vi "Append Multi Data Elements.vi"(8 "error in (no error)":errorcluster, 9 "Data Alias Array":string[](array[string]), 10 "Data Array":refnum<class "Data.lvclass">[](array[class]), 11 "Multi Data in":refnum<class "Multi Data.lvclass">) -> (0 "error out":errorcluster, 3 "Multi Data out":refnum<class "Multi Data.lvclass">)   [LabVIEW 2020, in "Publisher.lvlib" / "Multi Data.lvclass"]
doc: "Append Data and Data Alias Arrays to the arrays already stored on the class."
uses:
  Multi Data.lvclass
  PPL/HDH.Data.Generic.lvlibp/Data.lvclass
  Multi Data.lvclass/Multi Data.ctl
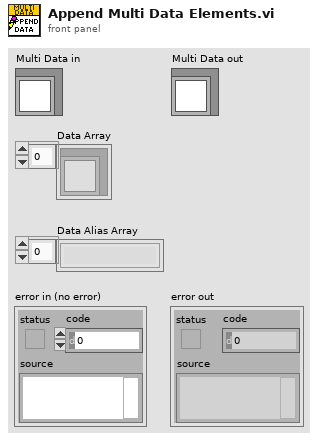
[diagram p1: front panel]
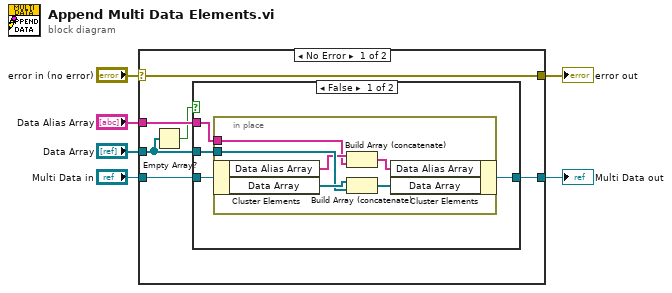
[diagram p0: block diagram]
diagram:
  n1 = case shown="No Error" "error in (no error)" {
    selector: "error in (no error)" -> [w12 w24]
    tunnel: [w12 w24] -> w5
    tunnel: [w10 w25] -> w3
    tunnel: "Multi Data in" -> [w11 w25]
    tunnel: "Data Array" -> [w8 _]
    tunnel: "Data Alias Array" -> [w9 _]
    frame No Error {
      n2 = Empty Array?(array=w8) -> (empty?=w7:bool)
      n3 = case shown="False" w7 {
        tunnel: w11 -> [w14 w23]
        tunnel: [w13 w23] -> w10
        tunnel: w9 -> [w16 _]
        tunnel: w8 -> [w15 _]
        frame False {
          n4 = in-place {
            in-place-border: w16 -> [w18]
            in-place-border: w15 -> [w21]
            n5 = in-place-cluster #1(w14) -> ("Data Alias Array"=w19:string[], "Data Array"=w22:refnum<class "Data.lvclass">[])
            n6 = Build Array (concatenate)(w19, w18) -> (w17:string[])
            n7 = Build Array (concatenate)(w22, w21) -> (w20:refnum<class "Data.lvclass">[])
            n8 = in-place-cluster #1("Data Alias Array"=w17, "Data Array"=w20) -> (w13:refnum<class "Multi Data.lvclass">)
          }
        }
        frame True {
        }
      }
    }
    frame Error {
    }
  }
  "error out" <- w5
  "Multi Data out" <- w3
